vi "Check if Bounce is Necessary.vi"(8 "error in":errorcluster, 11 "Display State In":T1 caption="State") -> (0 "error out":errorcluster, 2 "Was Bounce Done?":bool, 3 "Display State Out 2":T1={"Numeric"=0.0, "Array of Button References"=[], "Space Between Menu Buttons"=3, "Number of Menu Buttons"=6, "Array of Button Names"=[], "Most Recent Vertical Position"=0, "This VI"=refnum, "Current Action"=enum."Not Moving", "Most Recent Distance Traveled"=0, "Method"=enum."Resize", "Data In"=0} caption="State")   [LabVIEW 2011, in "Sliding Menu Library.lvlib" / "Sliding Menu XControl.xctl"]
uses:
  Sliding Menu xControl/Sliding Menu XControl.xctl
  Sliding Menu xControl/Sliding Menu State.ctl
  Menu Button Library/Menu Button xControl/Menu Button xControl.xctl
  Sliding Menu Type Definitions/Current User Action.ctl
  Sliding Menu xControl/Sliding Menu Methods.ctl
  Sliding Menu xControl/Sliding Menu Data.ctl
  Sliding Menu Library.lvlib
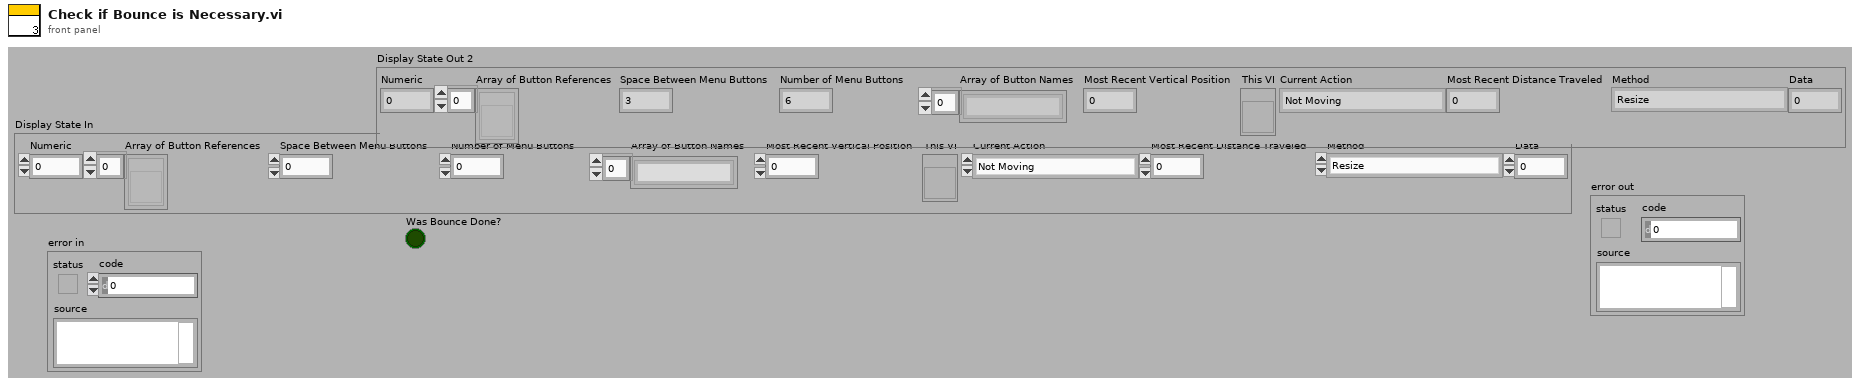
[diagram p1: front panel]
types:
  T1 = typedef "Sliding Menu Library.lvlib/Sliding Menu XControl.xctl/Sliding Menu State.ctl" = cluster{"Numeric":dbl, "Array of Button References":refnum<vi>[], "Space Between Menu Buttons":i32, "Number of Menu Buttons":i32, "Array of Button Names":string[], "Most Recent Vertical Position":i32, "This VI":refnum<vi>, "Current Action":T2, "Most Recent Distance Traveled":i32, "Method":T3, "Data In":T4}
  T2 = typedef "Sliding Menu Library.lvlib/Current User Action.ctl" = enum16{"Not Moving", "Mouse Down", "Mouse Up No Dragging", "Bounce Up Needed", "Bounce Down Needed", "Dragging", "Easing"}
  T3 = typedef "Sliding Menu Methods.ctl" = enum16{"Resize", "Move Up", "Move Down", "Move to 0"}
  T4 = typedef "Sliding Menu Library.lvlib/Sliding Menu XControl.xctl/Sliding Menu Data.ctl" = i32
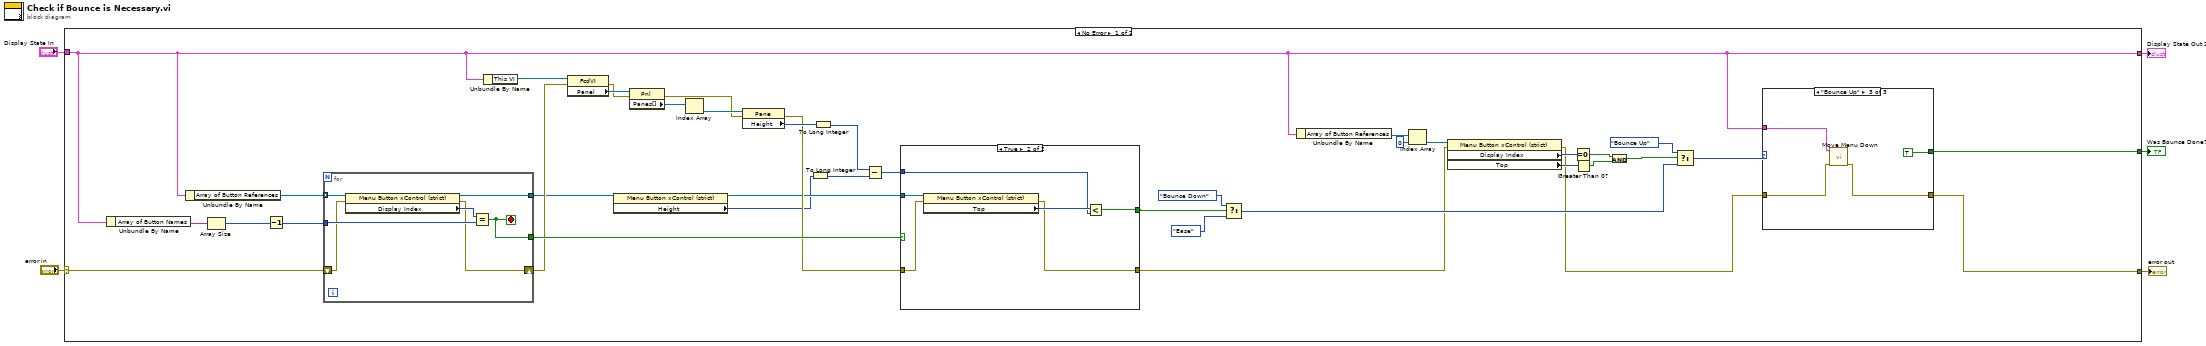
[diagram p0: block diagram]
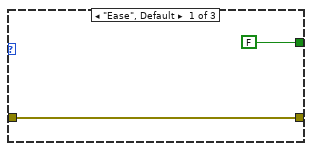
[diagram p2: hidden frame]
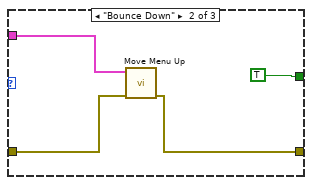
[diagram p3: hidden frame]
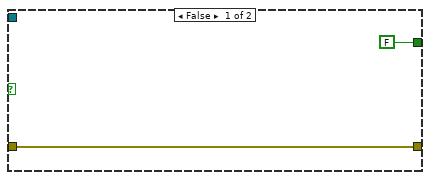
[diagram p4: hidden frame]
diagram:
  n1 = case shown="No Error" "error in" {
    selector: "error in" -> [w17 w71]
    tunnel: "Display State In" -> [w15 _]
    tunnel: [w13 w71] -> w5
    tunnel: [w15 _] -> w2
    tunnel: [w12 _] -> w1
    frame No Error {
      n2 = Unbundle By Name(w15) -> ("Array of Button Names"=w45:string[])
      n3 = Unbundle By Name(w15) -> ("Array of Button References"=w44:refnum<vi>[])
      n4 = Array Size(array=w45) -> (size(s)=w43:i32)
      n5 = Decrement(x=w43) -> (x-1=w42:i32)
      n6 = for {
        tunnel: w44 -> [w70] mode=indexing
        tunnel: w42 -> [w68]
        tunnel: [w67] -> w11
        shift-right: [w66] -> w21
        shift-left: w17 -> [w65]
        tunnel: [w64] -> w41
        stop <- w64 stop-if-true
        n7 = property class="Menu Button xControl (strict)"(reference=w70, error in=w65) -> (reference out=w67:refnum<vi>, error out=w66:errorcluster, "Display Index"=w69:i32)
        n8 = Equal?(x=w69, y=w68) -> (x = y?=w64:bool)
      }
      n9 = Unbundle By Name(w15) -> ("This VI"=w37:refnum<vi>)
      n10 = property class="FcdVI"(reference=w37, error in=w21) -> (error out=w20:errorcluster, "Panel"=w36:refnum<vi>)  [unwired: 1 out]
      n11 = property class="Menu Button xControl (strict)"(reference=w11) -> (reference out=w10:refnum<vi>, "Height"=w6:u32)  [unwired: 1 in, 1 out]
      n12 = property class="Pnl"(reference=w36, error in=w20) -> (error out=w19:errorcluster, "Panes[]"=w35:refnum<vi>[])  [unwired: 1 out]
      n13 = Index Array(array=w35) -> (element=w34:refnum<vi>)  [unwired: 1 in]
      n14 = property class="Pane"(reference=w34, error in=w19) -> (error out=w22:errorcluster, "Height"=w33:u32)  [unwired: 1 out]
      n15 = To Long Integer(number=w6) -> (32bit integer=w7:i32)
      n16 = To Long Integer(number=w33) -> (32bit integer=w9:i32)
      n17 = Subtract(x=w9, y=w7) -> (x-y=w8:i32)
      n18 = case shown="True" w41 {
        tunnel: w10 -> [_ w63]
        tunnel: w22 -> [w57 w61]
        tunnel: [w57 w60] -> w18
        tunnel: [FALSE w59] -> w38
        tunnel: w8 -> [_ w58]
        frame False {
        }
        frame True {
          n19 = property class="Menu Button xControl (strict)"(reference=w63, error in=w61) -> (error out=w60:errorcluster, "Top"=w62:i32)  [unwired: 1 out]
          n20 = Less?(x=w62, y=w58) -> (x < y?=w59:bool)
        }
      }
      n21 = Select(t=enum16{"Ease", "Bounce Down", "Bounce Up"}."Bounce Down" ("Enum"), s=w38, f=enum16{"Ease", "Bounce Down", "Bounce Up"}."Ease" ("Enum")) -> (s? t:f=w24:enum16{"Ease", "Bounce Down", "Bounce Up"})
      n22 = Unbundle By Name(w15) -> ("Array of Button References"=w32:refnum<vi>[])
      n23 = Index Array(array=w32, index=0) -> (element=w31:refnum<vi>)
      n24 = property class="Menu Button xControl (strict)"(reference=w31, error in=w18) -> (error out=w14:errorcluster, "Display Index"=w30:i32, "Top"=w29:i32)  [unwired: 1 out]
      n25 = Equal To 0?(x=w30) -> (x = 0?=w27:bool)
      n26 = Greater Than 0?(x=w29) -> (x > 0?=w26:bool)
      n27 = And(x=w27, y=w26) -> (x .and. y?=w25:bool)
      n28 = Select(t=enum16{"Ease", "Bounce Down", "Bounce Up"}."Bounce Up" ("Enum"), s=w25, f=w24) -> (s? t:f=w16:enum16{"Ease", "Bounce Down", "Bounce Up"})
      n29 = case shown="\"Bounce Up\"" w16 {
        tunnel: w14 -> [w47 w50 w54]
        tunnel: w15 -> [_ w51 w55]
        tunnel: [w47 w48 w53] -> w13
        tunnel: [FALSE TRUE TRUE] -> w12
        frame "Ease", Default {
        }
        frame "Bounce Down" {
          n30 = call "Move Menu Up.vi"("error in (no error)"=w50, "Display State In"=w51) -> ("error out"=w48:errorcluster)  [unwired: 8 in, 1 out]
        }
        frame "Bounce Up" {
          n31 = call "Move Menu Down.vi"("error in (no error)"=w54, "Display State In"=w55) -> ("error out"=w53:errorcluster)  [unwired: 8 in, 1 out]
        }
      }
    }
    frame Error {
    }
  }
  "error out" <- w5
  "Display State Out 2" <- w2
  "Was Bounce Done?" <- w1
